vi "Arm Extend Controller.vi"(1 "error in":errorcluster, 2 "Trigger":bool) -> (0 "error out":errorcluster)   [LabVIEW 2017]
uses:
  <vilib>/Rock Robotics/WPI/Solenoid/WPI_SolenoidValue.ctl
  Global Arm Variables.vi
  <vilib>/Rock Robotics/Network Tables/NT Write Boolean.vi
  <vilib>/Rock Robotics/WPI/Solenoid/WPI_SolenoidSetEnum.vi
panel:
  out "illegalRangeForExtendedArm":bool
  out "Command":T1
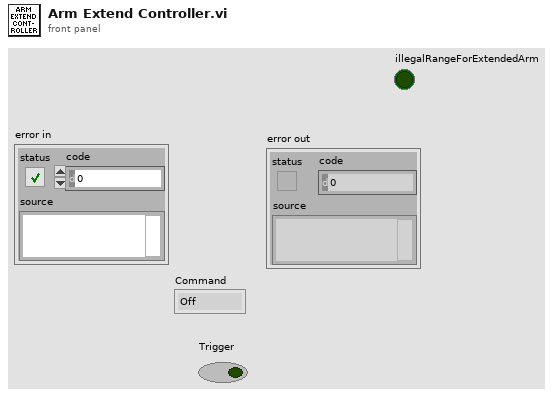
[diagram p1: front panel]
types:
  T1 = typedef "WPI_SolenoidValue.ctl" = enum16{"Off", "On", "Forward", "Reverse"}
  T2 = typedef "WPI_SolenoidDevRef.ctl" = cluster{"DevStatus":errorcluster, "Pneumatics Control Module":u8, "Forward Solenoid Channel":T3, "Reverse Solenoid Channel":T3}
  T3 = typedef "WPI_SolenoidChannel.ctl" = enum8{"Solenoid 0", "Solenoid 1", "Solenoid 2", "Solenoid 3", "Solenoid 4", "Solenoid 5", "Solenoid 6", "Solenoid 7", "Invalid"}
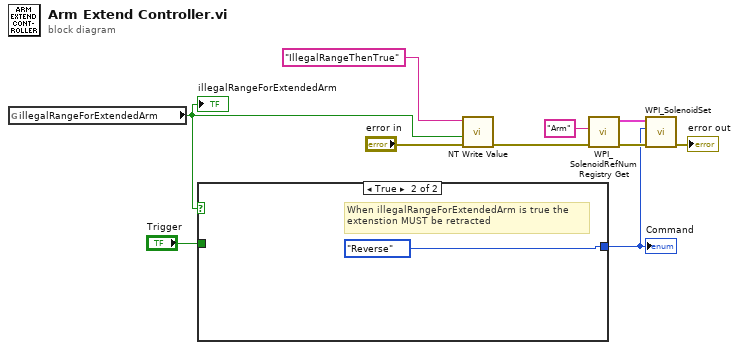
[diagram p0: block diagram]
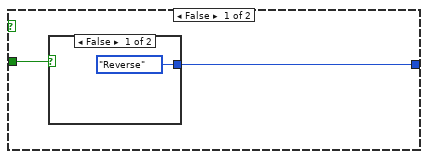
[diagram p2: hidden frame]
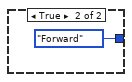
[diagram p3: hidden frame]
diagram:
  n1 = global read "Global Arm Variables.vi" "illegalRangeForExtendedArm"() -> (w3:bool)
  "illegalRangeForExtendedArm" <- w3
  n2 = case shown="True" w3 {
    tunnel: "Trigger" -> [w12 _]
    tunnel: [w11 WPI_SolenoidValue."Reverse" ("Value")] -> w5
    frame False {
      n3 = case shown="False" w12 {
        tunnel: [WPI_SolenoidValue."Reverse" ("Value") WPI_SolenoidValue."Forward" ("Value")] -> w11
        frame False {
        }
        frame True {
        }
      }
    }
    frame True {
      # "When illegalRangeForExtendedArm is true the\nextenstion MUST be retracted"
    }
  }
  "Command" <- w5
  n4 = call-poly <vilib>:"NT Write Value.vi"("error in"="error in", "Boolean"=w3, "Name"="IllegalRangeThenTrue") -> ("error out"=w1:errorcluster)  [unwired: 8 in]
  n5 = call <vilib>:"WPI_SolenoidRefNum Registry Get.vi"("error in (no error)"=w1, "refnum name"="Arm" ("Motor ID")) -> ("error out"=w7:errorcluster, "SolenoidDevRef"=w8:T2)  [unwired: 8 in]
  n6 = call-poly <vilib>:"WPI_SolenoidSet.vi"("error in (no error)"=w7, "Value"=w5, "SolenoidDevRef"=w8) -> ("error out"=→"error out":errorcluster)  [unwired: 7 in, 1 out]
